vi "MS Close.vi"(8 "error in (no error)":errorcluster, 10 "VISA Refnum in 2":refnum<visa-resource-name>, 11 "VISA Refnum in":refnum<visa-resource-name>) -> (0 "error out":errorcluster)   [LabVIEW 2012]
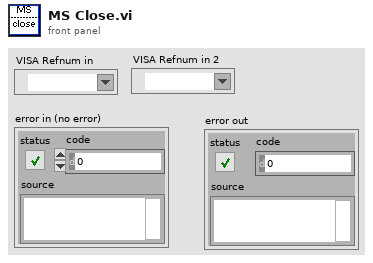
[diagram p1: front panel]
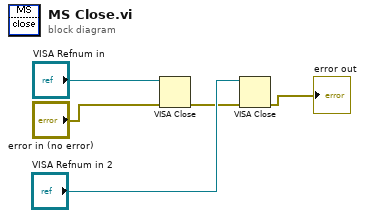
[diagram p0: block diagram]
diagram:
  n1 = VISA Close(VISA resource name="VISA Refnum in", error in (no error)="error in (no error)") -> (error out=w2:errorcluster)
  n2 = VISA Close(VISA resource name="VISA Refnum in 2", error in (no error)=w2) -> (error out=→"error out":errorcluster)
